vi "TCPClient.vi"() -> ()   [LabVIEW 2014]
uses:
  Global/ClientGlobalCY.vi
  CYY/cyy.lvlib
  LeakageFenxi/LeakageFenXi.lvlib
panel:
  in  "quit":bool
  in  "获取区域信息":bool
  in  "获取采样数据信息":bool
  in  "选项卡控件":enum32{"数据监测界面", "选项卡 2"}(tab)
  in  "数据监测界面":i32(listbox)
  out "区域信息":string[][](array[string])
  out "采样数据":string[][](array[string])
  out "error out":errorcluster caption="错误输出"
  in  "error in (no error)":errorcluster caption="错误输入（无错误）"
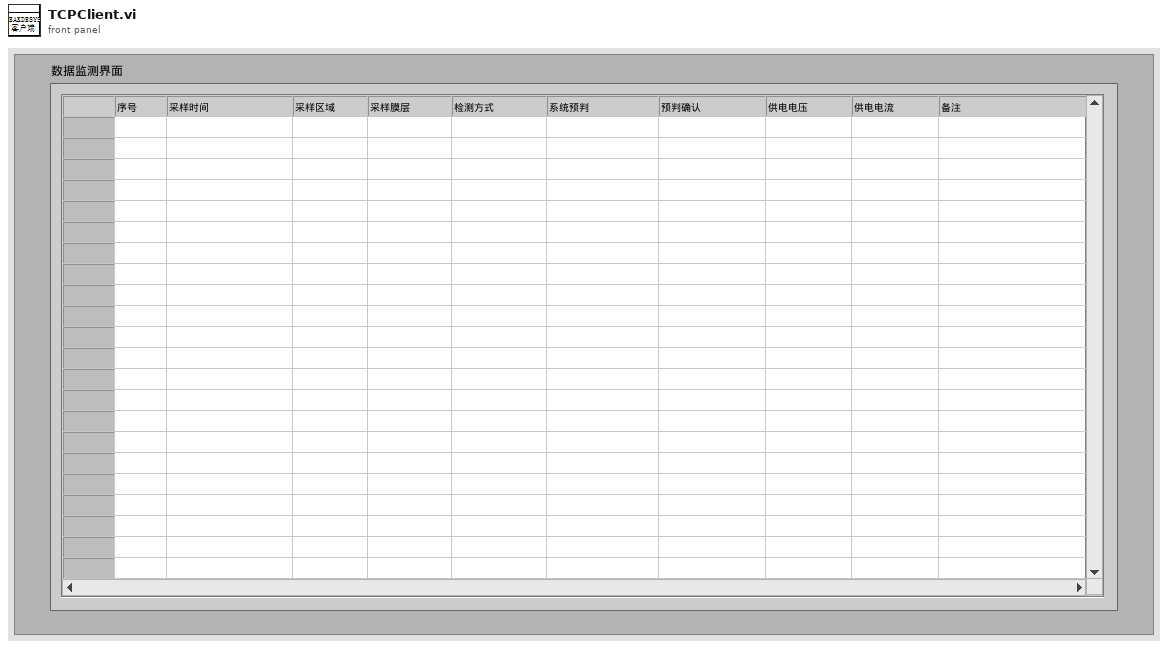
[diagram p1: front panel]
types:
  T1 = enum32{"invalid app kind", "Development System", "Run Time System", "Student Edition", "Embedded LabVIEW", "Evaluation", "Custom"}
  T2 = enum32{"Invalid", "Standard", "Closed", "Hidden", "Minimized", "Maximized"}
  T3 = cluster{"Core":cluster{"Current VI Reference":refnum<vi>, "Close Panel on Exit?":bool}, "Your Boolean data":bool, "Your string data":string, "connectionID":refnum<k5>, "Row":i32, "SampleInfoTime":string, "AreaName":string, "采样数据":string[][], "是否存在记录？":bool}
  T4 = typedef "LVPoint32TypeDef.ctl" = cluster{"Horizontal":i32, "Vertical":i32}
  T5 = typedef "LVRowAndColumnTypeDef.ctl" = cluster{"Row":i32, "Column":i32}
  T6 = typedef "LVRectTypeDef.ctl" = cluster{"Left":i16, "Top":i16, "Right":i16, "Bottom":i16}
  T7 = cluster{"Current VI Reference":refnum<vi>, "Close Panel on Exit?":bool}
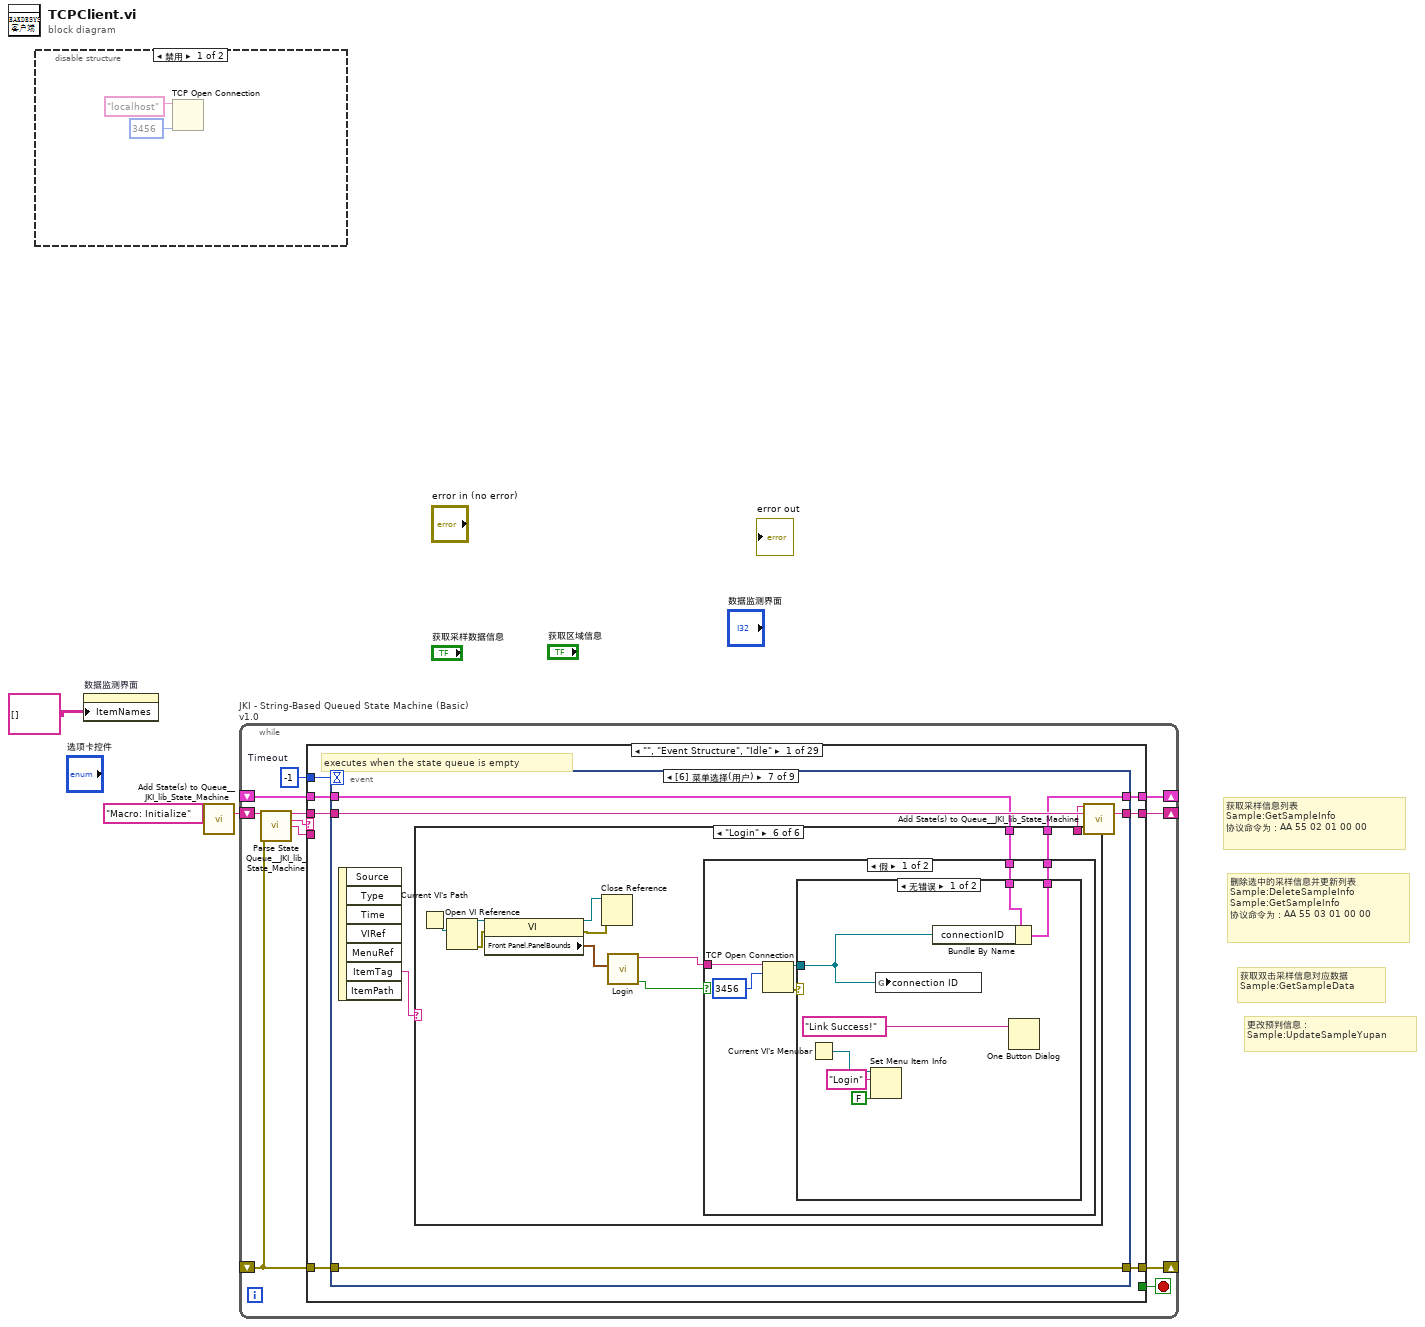
[diagram p0: block diagram]
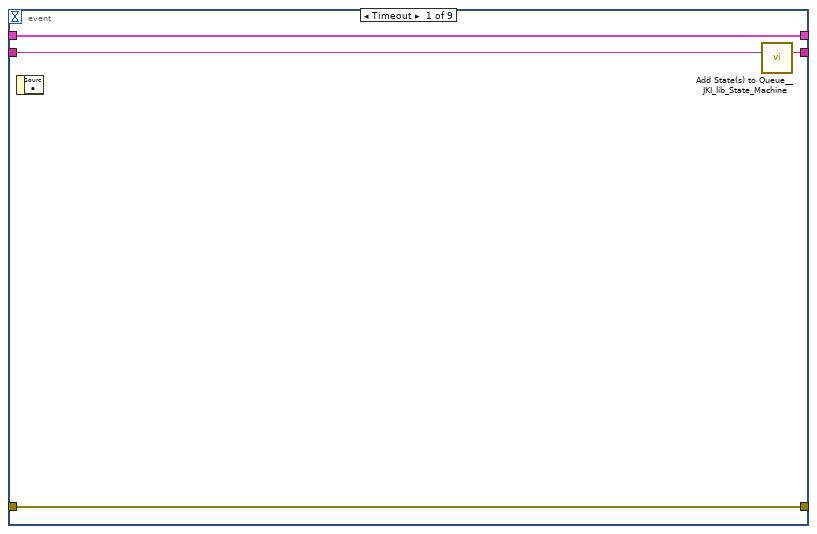
[diagram p3: hidden frame]
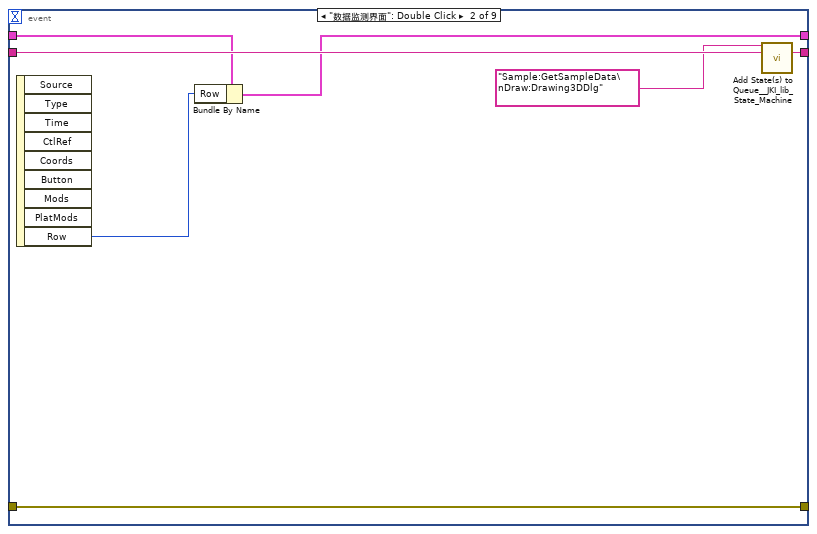
[diagram p4: hidden frame]
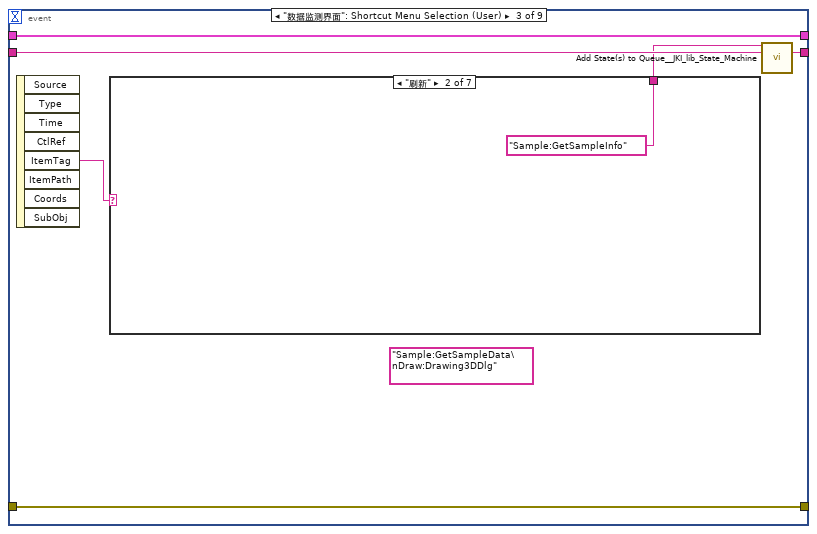
[diagram p5: hidden frame]
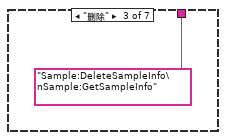
[diagram p7: hidden frame]
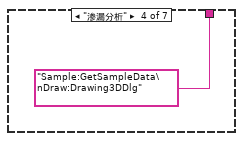
[diagram p8: hidden frame]
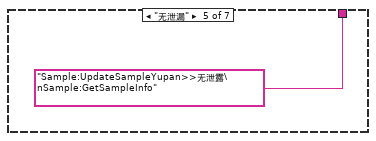
[diagram p9: hidden frame]
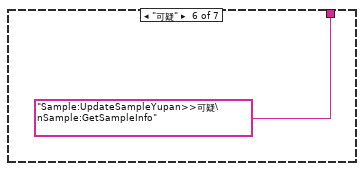
[diagram p10: hidden frame]
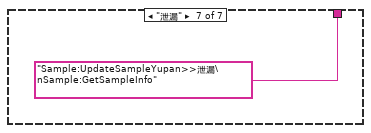
[diagram p11: hidden frame]
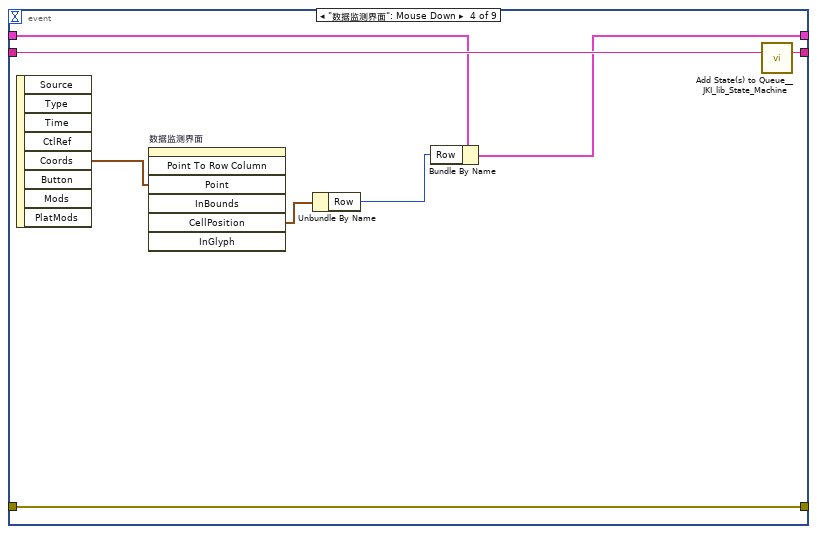
[diagram p12: hidden frame]
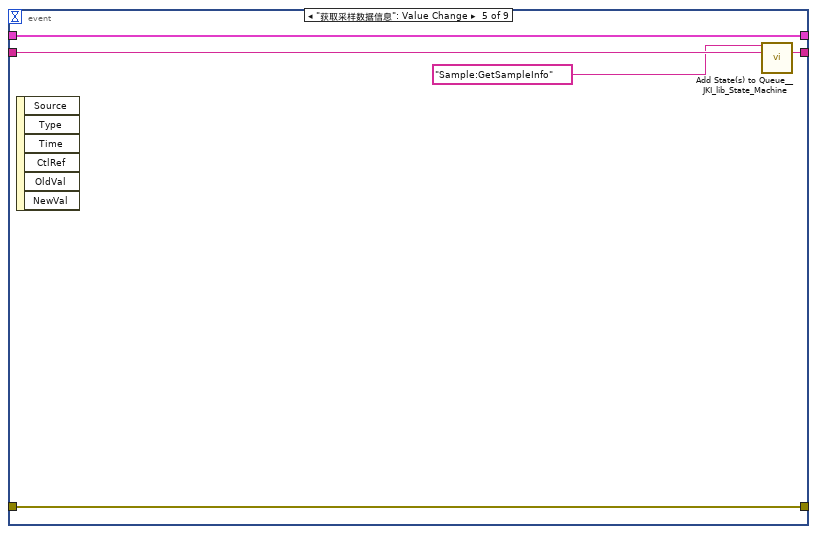
[diagram p13: hidden frame]
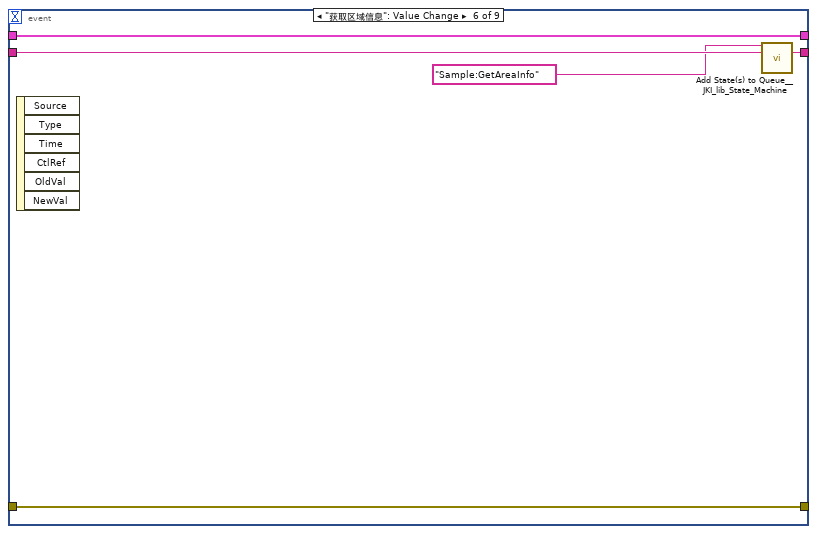
[diagram p14: hidden frame]
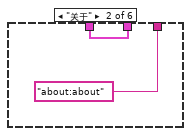
[diagram p16: hidden frame]
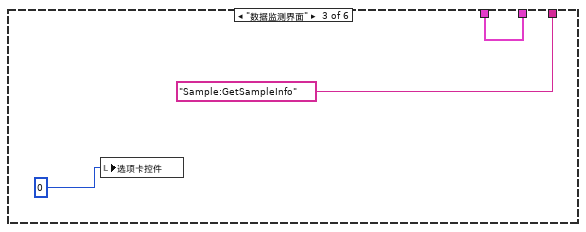
[diagram p17: hidden frame]
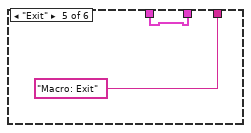
[diagram p19: hidden frame]
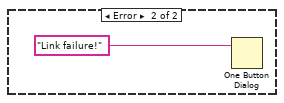
[diagram p20: hidden frame]
diagram:
  # "更改预判信息：\nSample:UpdateSampleYupan"
  # "获取双击采样信息对应数据\nSample:GetSampleData"
  # "删除选中的采样信息并更新列表\nSample:DeleteSampleInfo\nSample:GetSampleInfo\n协议命令为：AA 55 03 01 00 00"
  # "获取采样信息列表\nSample:GetSampleInfo\n协议命令为：AA 55 02 01 00 00"
  n1 = disable-structure shown="禁用" {
    frame Disabled {
      n2 = TCP Open Connection(address="localhost" ("地址"), remote port or service name=u16 3456 ("远程端口或服务名称")) -> ()  [unwired: 3 in, 2 out]
    }
    frame Enabled {
    }
  }
  n3 = property on="数据监测界面" class="MCListbox (严格)"("ItemNames"=string[][] []) -> ()  [unwired: 2 in, 2 out]
  n4 = call <vilib>:"Add State(s) to Queue__JKI_lib_State_Machine.vi"("State(s) in (\"\")"="Macro: Initialize") -> ("States Out"=w3:string)  [unwired: 14 in]
  n5 = while "JKI - String-Based Queued State Machine (Basic) v1.0" {
    shift-right: [w9] -> _
    shift-left: _ -> [w8]
    shift-right: [w12] -> _
    shift-left: _ -> [w6]
    shift-right: [w11] -> _
    shift-left: w3 -> [w13]
    stop <- w10 stop-if-true
    w7 = -1  # Timeout
    n6 = call <vilib>:"Parse State Queue__JKI_lib_State_Machine.vi"("State Queue"=w13, "Error In (no error)"=w6) -> ("Remaining States"=w15:string, "Current State"=w16:string, "Arguments"=w14:string)  [unwired: 11 in]
    n7 = case shown="\"\", \"Event Structure\", \"Idle\"" w16 {
      selector: w16 -> [_ _ w118 _ _ _ _ _ _ _ _ _ _ _ _ _ _ _ _ _ _ _ _ _ _ _ _ _ _]
      tunnel: w15 -> [w23 w117 w122 w140 w146 w151 w155 w168 w174 w178 w182 w188 w199 w225 w230 w240 w244 w248 w252 w256 w260 w264 w272 w276 w291 w308 w320 w327 w334]
      tunnel: w14 -> [_ _ _ _ _ _ _ _ _ _ _ w183 w193 _ _ _ _ _ _ _ _ _ _ _ w280 _ _ _ _]
      tunnel: w8 -> [w21 w114 w120 w131 w143 w149 w152 _ w169 w175 w180 w186 w195 w222 w227 w237 w241 w245 w249 w253 w257 w261 w269 w273 w288 w298 w317 w325 w330]
      tunnel: [w20 w115 w124 w137 errorcluster {"status"=FALSE, "code"=0, "source"=""} ("error out") w148 w153 w165 w170 w176 w179 w184 w196 w223 w228 w238 w242 w246 w250 w254 w258 w262 w270 w274 w289 w306 w318 w322 w331] -> w12
      tunnel: w6 -> [w19 w115 w123 w137 w142 w148 w153 w165 w171 w176 w179 w185 w197 w223 w228 w238 w242 w246 w250 w254 w258 w262 w270 w274 w289 w306 w318 w323 w332]
      tunnel: [w22 w116 w121 w139 w145 w150 w154 w167 w173 w177 w181 w187 w198 w224 w229 w239 w243 w247 w251 w255 w259 w263 w271 w275 w290 w307 w319 w326 w333] -> w11
      tunnel: [_ _ _ _ _ TRUE _ _ _ _ _ _ _ _ _ _ _ _ _ _ _ _ _ _ _ _ _ _ _] -> w10
      tunnel: [w18 w114 w120 w138 w143 w149 w152 w166 w169 w175 w180 w186 w195 w222 w227 w237 w241 w245 w249 w253 w257 w261 w269 w273 w288 w297 w317 w325 w330] -> w9
      tunnel: w7 -> [w17 _ _ _ _ _ _ _ _ _ _ _ _ _ _ _ _ _ _ _ _ _ _ _ _ _ _ _ _]
      frame "", "Event Structure", "Idle" {
        # "executes when the state queue is empty"
        n8 = event shown="[6] 菜单选择(用户)" {
          selector: _ -> [_ _ _ _ _ _ _ _ _]
          dyn-events: _ -> [_ _ _ _ _ _ _ _ _]
          timeout: w17 -> [_ _ _ _ _ _ _ _ _]
          tunnel: w23 -> [w27 w34 w40 w54 w59 w64 w71 w107 w113]
          tunnel: [w26 w33 w39 w53 w58 w63 w70 w106 w112] -> w22
          tunnel: w21 -> [w24 w31 w37 w48 w56 w61 w67 w104 w110]
          tunnel: [w25 w32 w38 w52 w57 w62 w69 w105 w111] -> w20
          tunnel: w19 -> [w25 w32 w38 w52 w57 w62 w69 w105 w111]
          tunnel: [w24 w28 w37 w47 w56 w61 w66 w104 w110] -> w18
          event Timeout {
            n9 = event-data() -> ()  [unwired: 1 in, 1 out]
            n10 = call <vilib>:"Add State(s) to Queue__JKI_lib_State_Machine.vi"("State(s) in (\"\")"=w27) -> ("States Out"=w26:string)  [unwired: 14 in]
          }
          event "数据监测界面": Double Click {
            n11 = event-data() -> ("Row"=w30:i32)  [unwired: 1 in, 8 out]
            n12 = Bundle By Name(cluster=w31, "Row"=w30) -> (w28:T3)
            n13 = call <vilib>:"Add State(s) to Queue__JKI_lib_State_Machine.vi"("State(s) in Front (\"\")"="Sample:GetSampleData\nDraw:Drawing3DDlg", "State(s) in (\"\")"=w34) -> ("States Out"=w33:string)  [unwired: 13 in]
          }
          event "数据监测界面": Shortcut Menu Selection (User) {
            (unwired) "Sample:GetSampleData\nDraw:Drawing3DDlg"
            n14 = event-data() -> ("ItemTag"=w36:string)  [unwired: 1 in, 7 out]
            n15 = case shown="\"刷新\"" w36 {
              tunnel: [_ "Sample:GetSampleInfo" "Sample:DeleteSampleInfo\nSample:GetSampleInfo" "Sample:GetSampleData\nDraw:Drawing3DDlg" "Sample:UpdateSampleYupan>>无泄露\nSample:GetSampleInfo" "Sample:UpdateSampleYupan>>可疑\nSample:GetSampleInfo" "Sample:UpdateSampleYupan>>泄漏\nSample:GetSampleInfo"] -> w35
              frame "假", Default {
              }
              frame "刷新" {
              }
              frame "删除" {
              }
              frame "渗漏分析" {
              }
              frame "无泄漏" {
              }
              frame "可疑" {
              }
              frame "泄漏" {
              }
            }
            n16 = call <vilib>:"Add State(s) to Queue__JKI_lib_State_Machine.vi"("State(s) in Front (\"\")"=w35, "State(s) in (\"\")"=w40) -> ("States Out"=w39:string)  [unwired: 13 in]
          }
          event "数据监测界面": Mouse Down {
            n17 = event-data() -> ("Coords"=w51:T4)  [unwired: 1 in, 7 out]
            n18 = invoke on="数据监测界面" class="MCListbox (严格)" method="Point To Row Column"("Point"=w51) -> ("CellPosition"=w50:T5)  [unwired: 6 in, 6 out]
            n19 = Unbundle By Name(w50) -> ("Row"=w49:i32)
            n20 = Bundle By Name(cluster=w48, "Row"=w49) -> (w47:T3)
            n21 = call <vilib>:"Add State(s) to Queue__JKI_lib_State_Machine.vi"("State(s) in (\"\")"=w54) -> ("States Out"=w53:string)  [unwired: 14 in]
          }
          event "获取采样数据信息": Value Change {
            n22 = event-data() -> ()  [unwired: 1 in, 6 out]
            n23 = call <vilib>:"Add State(s) to Queue__JKI_lib_State_Machine.vi"("State(s) in Front (\"\")"="Sample:GetSampleInfo", "State(s) in (\"\")"=w59) -> ("States Out"=w58:string)  [unwired: 13 in]
          }
          event "获取区域信息": Value Change {
            n24 = event-data() -> ()  [unwired: 1 in, 6 out]
            n25 = call <vilib>:"Add State(s) to Queue__JKI_lib_State_Machine.vi"("State(s) in Front (\"\")"="Sample:GetAreaInfo", "State(s) in (\"\")"=w64) -> ("States Out"=w63:string)  [unwired: 13 in]
          }
          event Menu Selection (User) {
            n26 = event-data() -> ("ItemTag"=w68:string)  [unwired: 1 in, 6 out]
            n27 = case shown="\"Login\"" w68 {
              tunnel: w67 -> [_ w73 w75 _ w78 w80]
              tunnel: [_ w73 w75 _ w78 w79] -> w66
              tunnel: [_ "about:about" "Sample:GetSampleInfo" _ "Macro: Exit" _] -> w65
              frame "假", Default {
              }
              frame "关于" {
              }
              frame "数据监测界面" {
                n28 = local write "选项卡控件"(0) -> ()
              }
              frame "Logout" {
              }
              frame "Exit" {
              }
              frame "Login" {
                n29 = Current VI's Path() -> (path=w88:path)
                n30 = Open VI Reference(vi path=w88) -> (vi reference=w87:refnum<vi>, error out=w86:errorcluster)  [unwired: 5 in]
                n31 = property class="VI"(reference=w87, error in=w86) -> (reference out=w84:refnum<vi>, error out=w85:errorcluster, "Front Panel.PanelBounds"=w83:T6)
                n32 = Close Reference(reference=w84, error in (no error)=w85) -> ()  [unwired: 1 out]
                n33 = call "Login.vi"("窗口边界"=w83) -> ("drop?"=w82:bool, "User IP"=w81:string)  [unwired: 8 in, 1 out]
                n34 = case shown="假" w82 {
                  tunnel: w81 -> [w94 _]
                  tunnel: w80 -> [w90 _]
                  tunnel: [w89 _] -> w79
                  frame False {
                    n35 = TCP Open Connection(address=w94, remote port or service name=u16 3456 ("远程端口或服务名称")) -> (connection ID=w91:refnum<k5>, error out=w92:errorcluster)  [unwired: 3 in]
                    n36 = case shown="无错误" w92 {
                      tunnel: w91 -> [w95 _]
                      tunnel: w90 -> [w97 _]
                      tunnel: [w96 _] -> w89
                      frame No Error {
                        n37 = Current VI's Menubar() -> (w101:refnum<k9>)
                        n38 = Set Menu Item Info(7:"Login" ("项名称"), 9:FALSE ("已启用"), 11:w101) -> ()  [unwired: 4 in, 2 out]
                        n39 = global write "ClientGlobalCY.vi" "connection ID"(w95) -> ()
                        n40 = Bundle By Name(cluster=w97, "connectionID"=w95) -> (w96:T3)
                        n41 = One Button Dialog(message="Link Success!" ("消息")) -> ()  [unwired: 1 in, 1 out]
                      }
                      frame Error {
                        n42 = One Button Dialog(message="Link failure!" ("消息")) -> ()  [unwired: 1 in, 1 out]
                      }
                    }
                  }
                  frame True {
                  }
                }
              }
            }
            n43 = call <vilib>:"Add State(s) to Queue__JKI_lib_State_Machine.vi"("State(s) in Front (\"\")"=w65, "State(s) in (\"\")"=w71) -> ("States Out"=w70:string)  [unwired: 13 in]
          }
          event "quit": Value Change {
            n44 = event-data() -> ()  [unwired: 1 in, 1 out]
            n45 = call <vilib>:"Add State(s) to Queue__JKI_lib_State_Machine.vi"("State(s) in Front (\"\")"="Macro: Exit", "State(s) in (\"\")"=w107) -> ("States Out"=w106:string)  [unwired: 13 in]
          }
          event Panel Close? {
            # "Discard the event because we'll close the front panel ourselves in Macro: Exit"
            # "Close Panel button (pressed) Event\n(this executes Macro: Exit to terminate the VI)"
            n46 = event-data() -> ()  [unwired: 1 in, 1 out]
            n47 = event-data("Discard?"=TRUE) -> ()  [unwired: 1 in, 1 out]
            n48 = call <vilib>:"Add State(s) to Queue__JKI_lib_State_Machine.vi"("State(s) in Front (\"\")"="Macro: Exit", "State(s) in (\"\")"=w113) -> ("States Out"=w112:string)  [unwired: 13 in]
          }
        }
      }
      frame "---------- Core ----------" {
        # "Do not put any code in this frame.\n(it is a separator no-op)"
        n49 = call <vilib>:"Add State(s) to Queue__JKI_lib_State_Machine.vi"("State(s) in (\"\")"=w117) -> ("States Out"=w116:string)  [unwired: 14 in]
      }
      frame Default {
        w127 = 42 items=["No error", "Argument error", "Memory is full", "Out of zone", "End of file", "File already open", "Generic file I/O error", "File not found", "File permission error", "Disk is full", "Duplicate path", "Too many files open", "System feature not enabled", "Resource file not found", "Cannot add resource", "Resource not found", "Image not found", "Image memory error", "Pen does not exist", "Config type invalid", "Config token not found", "Config parse error", "Config memory error", "Bad external code format", "Bad external code offset", "External code not present", "Null window", "Destroy window error", "Null menu", "Print aborted", "Bad print record", "Print driver error", "Windows error during printing", "Memory error during printing", "Print dialog error", "Generic print error", "Invalid device refnum", "Device not found", "Device parameter error", "Device unit error", "Cannot open device", "Device call aborted", "Generic error", "Cancelled by user", "Object ID too low", "Object ID too high", "Object not in heap", "Unknown heap", "Unknown object (invalid DefProc)", "Unknown object (DefProc not in table)", "Message out of range", "Invalid (null) method", "Unknown message", "Manager call not supported", "Bad address", "Network operation in progress", "Network operation timed out", "Connection is busy", "Network attribute not supported", "Network error", "Address in use", "System out of memory", "Connection aborted", "Connection refused", "Not connected", "Already connected", "Connection closed", "Initialization error (interapplication manager)", "Bad occurrence", "Wait on unbound occurrence handler", "Occurrence queue overflow", "Datalog type conflict", "Unused", "Unrecognized type (interapplication manager)", "Memory corrupt", "Failed to make temporary DLL", "Old CIN version", "Drag socket not found", "Failed to load drop-object", "Failed to register OLE object", "Failed to release OLE object", "Format specifier type mismatch", "Unknown format specifier", "Too few format specifiers", "Too many format specifiers", "Scan failed", "Newer CIN version", "Error converting to variant", "Runtime menu error", "Password tampered", "Variant attribute not found", "Incompatible variant data type", "Event data is not available", "Event Store is not present", "Occurrence is not found", "Event Queue is not created", "Event info is not available", "Refnum passed is NULL", "Error retrieving Class GUID", "Error retrieving CoClass GUID", "Error retrieving TypeLib GUID.", "Bad built application magic bytes.", "Specific driver is different from the specific driver associated with the Logical Name.", "There is no session opened to the class driver.", "Max Error", "MAX - Error with config objects", "MAX - Error loading configuration", "MAX - Group not supported"]
        # "Current State"
        # "Do not delete, rename, or modify this frame.\n(this is used to capture unhandled states and typos)"
        # "Handle mistyped state name (developer tool)"
        n50 = Format Into String(format string="Software Exception: Unhandled State \"%s\"." ("message"), error in=w123, w118) -> (resulting string=w126:string, error out=w125:errorcluster)  [unwired: 1 in]
        n51 = call <vilib>:"Error Cluster From Error Code.vi"("show call chain? (False)"=TRUE, "error in (no error)"=w125, "error message (\"\")"=w126, "error code (0)"=w127) -> ("error out"=w124:errorcluster)  [unwired: 5 in]
        n52 = call <vilib>:"Add State(s) to Queue__JKI_lib_State_Machine.vi"("State(s) in (\"\")"=w122) -> ("States Out"=w121:string)  [unwired: 14 in]
      }
      frame "Initialize Core Data" {
        # "Do not delete, rename, or modify this frame.\n(this is used to determine panel behavior on exit)"
        # "originally closed?"
        # "exe?"
        # "If panel starts closed or is an EXE, then close it when we exit"
        n53 = property class="VI"() -> ("Front Panel.Open"=w136:bool)  [unwired: 2 in, 2 out]
        n54 = property class="App"() -> ("App.Kind"=w135:T1)  [unwired: 2 in, 2 out]
        n55 = control-ref of="Current VI Reference"() -> (w129:refnum<vi>)
        n56 = Not(x=w136) -> (.not. x?=w133:bool)
        n57 = Equal?(x=w135, y=T1."Run Time System" ("Application:Kind")) -> (x = y?=w132:bool)
        n58 = Or(x=w133, y=w132) -> (x .or. y?=w130:bool)
        n59 = Bundle By Name(cluster=w131, "Core.Current VI Reference"=w129, "Core.Close Panel on Exit?"=w130) -> (w138:T3)
        n60 = call <vilib>:"Add State(s) to Queue__JKI_lib_State_Machine.vi"("State(s) in (\"\")"=w140) -> ("States Out"=w139:string)  [unwired: 14 in]
      }
      frame "Error Handler" {
        # "Unhandled Error -- Display it"
        # "Handle any errors here.\nYou can also output any states to clean-up after errors occur"
        # "Clear error"
        n61 = call <vilib>:"General Error Handler.vi"("error in (no error)"=w142) -> ()  [unwired: 10 in, 5 out]
        n62 = call <vilib>:"Add State(s) to Queue__JKI_lib_State_Machine.vi"("State(s) in Front (\"\")"="/* Post Error States", "State(s) in (\"\")"=w146) -> ("States Out"=w145:string)  [unwired: 13 in]
      }
      frame "Exit" {
        # "Do not put any code in this frame.\n(No errors that occur here will be handled.)"
        n63 = call <vilib>:"Add State(s) to Queue__JKI_lib_State_Machine.vi"("State(s) in (\"\")"=w151) -> ("States Out"=w150:string)  [unwired: 14 in]
      }
      frame "---------- Data ----------" {
        # "Do not put any code in this frame.\n(It is a separator no-op. You can make a copy of this frame to create a new Data frame)"
        n64 = call <vilib>:"Add State(s) to Queue__JKI_lib_State_Machine.vi"("State(s) in (\"\")"=w155) -> ("States Out"=w154:string)  [unwired: 14 in]
      }
      frame "Data: Initialize" {
        w156 = TRUE  # 是否存在记录？
        w158 = ""  # AreaName
        w159 = ""  # SampleInfoTime
        w160 = 0  # Row
        w161 = refnum<k5> refnum  # connectionID
        w162 = T7 {"Current VI Reference"=refnum, "Close Panel on Exit?"=FALSE}  # Core
        w164 = TRUE  # Your Boolean data
        w163 = ""  # Your string data
        # "do not delete - used by framework"
        # "Data names and types of shift register data are defined by this bundle."
        # "Initialize the shift-register data, here.\n(data names are defined by what you wire into the bundle function)"
        n65 = Bundle("Core"=w162, "Your Boolean data"=w164, "Your string data"=w163, "connectionID"=w161, "Row"=w160, "SampleInfoTime"=w159, "AreaName"=w158, "采样数据"=string[][] [["101", "39", "0", "9.701"], ["102", "37", "0", "9.699"], ["103", "40", "2", "9.699"], ["104", "38", "2", "9.696"], ["105", "36", "2", "9.698"], ["106", "41", "4", "9.708"], ["107", "39", "4", "9.699"], ["108", "37", "4", "9.702"], ["109", "35", "4", "9.703"], ["110", "40", "6", "9.698"], ["111", "36", "6", "9.690"], ["112", "41", "8", "9.707"], ["113", "39", "8", "9.705"], ["114", "37", "8", "9.694"], ["115", "35", "8", "9.698"], ["116", "40", "10", "9.702"], ["117", "38", "10", "9.703"], ["118", "36", "10", "9.699"], ["119", "34", "10", "9.700"], ["120", "39", "12", "9.704"], ["121", "37", "12", "9.699"], ["122", "40", "14", "9.700"], ["123", "38", "14", "9.699"], ["124", "36", "14", "9.699"], ["125", "41", "16", "9.699"], ["126", "39", "16", "9.698"], ["127", "37", "16", "9.701"], ["128", "35", "16", "9.696"], ["129", "40", "18", "9.697"], ["130", "36", "17.75", "9.698"], ["131", "70", "0", "9.701"], ["132", "60", "0", "9.700"], ["133", "50", "0", "9.701"], ["134", "40", "8", "9.699"], ["135", "32", "8", "9.699"], ["136", "40", "0", "9.696"], ["137", "32", "0", "9.698"], ["138", "40", "8", "9.708"], ["139", "32", "8", "9.699"], ["140", "40", "0", "9.702"], ["141", "70", "0", "9.703"], ["142", "60", "0", "9.698"], ["201", "33", "0", "9.690"], ["202", "31", "0", "9.707"], ["203", "34", "2", "9.705"], ["204", "32", "2", "9.694"], ["205", "30", "2", "9.698"], ["206", "28", "2", "9.702"], ["207", "33", "4", "9.703"], ["208", "31", "4", "9.699"], ["209", "29", "4", "9.700"], ["210", "27", "4", "9.704"], ["211", "34", "6", "9.699"], ["212", "30", "6", "9.700"], ["213", "28", "6", "9.699"], ["214", "33", "8", "9.699"], ["215", "31", "8", "9.699"], ["216", "29", "8", "9.698"], ["217", "27", "8", "9.701"], ["218", "32", "10", "9.696"], ["219", "30", "10", "9.697"], ["220", "28", "10", "9.698"], ["221", "33", "12", "9.701"], ["222", "31", "12", "9.700"], ["223", "34", "14", "9.701"], ["224", "32", "14", "9.699"], ["225", "30", "14", "9.699"], ["226", "28", "14", "9.696"], ["227", "33", "16", "9.698"], ["228", "31", "16", "9.708"], ["229", "29", "16", "9.699"], ["230", "34", "17.5", "9.702"], ["231", "30", "17", "9.703"], ["232", "28", "17", "9.698"], ["233", "40", "0", "9.690"], ["234", "30", "0", "9.707"], ["235", "24", "8", "9.705"], ["236", "16", "8", "9.694"], ["237", "24", "0", "9.698"], ["238", "16", "0", "9.702"], ["239", "24", "8", "9.703"], ["240", "32", "0", "9.699"], ["241", "24", "0", "9.700"], ["242", "16", "0", "9.704"], ["243", "50", "0", "9.699"], ["244", "40", "0", "9.700"], ["245", "30", "0", "9.699"], ["301", "27", "0", "9.699"], ["302", "25", "0", "9.699"], ["303", "21", "0", "9.698"], ["304", "19", "0", "9.701"], ["305", "26", "2", "9.696"], ["306", "24", "2", "9.697"], ["307", "22", "2", "9.698"], ["308", "20", "2", "9.701"], ["309", "18", "2", "9.700"], ["310", "25", "4", "9.701"], ["311", "23", "4", "9.699"], ["312", "21", "4", "9.699"], ["313", "19", "4", "9.696"], ["314", "17", "4", "9.698"], ["315", "24", "6", "9.708"], ["316", "22", "6", "9.699"], ["317", "18", "6", "9.702"], ["318", "25", "8", "9.703"], ["319", "23", "8", "9.698"], ["320", "21", "8", "9.690"], ["321", "19", "8", "9.707"], ["322", "26", "10", "9.705"], ["323", "24", "10", "9.694"], ["324", "22", "10", "9.698"], ["325", "20", "10", "9.702"], ["326", "18", "10", "9.703"], ["327", "27", "12", "9.699"], ["328", "25", "12", "9.700"], ["329", "21", "12", "9.704"], ["330", "19", "12", "9.699"], ["331", "26", "14", "9.700"], ["332", "24", "14", "9.699"], ["333", "22", "14", "9.699"], ["334", "20", "14", "9.699"], ["335", "27", "16", "9.698"], ["336", "25", "16", "9.701"], ["337", "23", "16", "9.696"], ["338", "21", "16", "9.697"], ["339", "19", "16", "9.698"], ["340", "24", "17", "9.701"], ["341", "22", "17", "9.700"], ["342", "18", "17.5", "9.701"], ["401", "15", "0", "9.699"], ["402", "13", "0", "9.699"], ["403", "16", "2", "9.696"], ["404", "14", "2", "9.698"], ["405", "12", "2", "9.708"], ["406", "15", "4", "9.699"], ["407", "13", "4", "9.702"], ["408", "11", "4", "9.703"], ["409", "16", "6", "9.698"], ["410", "12", "6", "9.690"], ["411", "47", "8", "9.707"], ["412", "15", "8", "9.705"], ["413", "13", "8", "9.694"], ["414", "11", "8", "9.698"], ["415", "16", "10", "9.702"], ["416", "14", "10", "9.703"], ["417", "12", "10", "9.699"], ["418", "10", "10", "9.700"], ["419", "15", "12", "9.704"], ["420", "13", "12", "9.699"], ["421", "18", "14", "9.700"], ["422", "16", "14", "9.699"], ["423", "14", "14", "9.699"], ["424", "12", "14", "9.699"], ["425", "17", "16", "9.698"], ["426", "15", "16", "9.701"], ["427", "13", "16", "9.696"], ["428", "16", "17.5", "9.697"], ["429", "12", "18", "9.698"], ["430", "10", "18", "9.701"], ["431", "30", "0", "9.700"], ["432", "20", "0", "9.701"], ["433", "0", "0", "9.699"], ["434", "8", "0", "9.699"], ["435", "0", "0", "9.696"], ["436", "16", "8", "9.698"], ["437", "8", "8", "9.708"], ["438", "0", "8", "9.699"], ["439", "20", "0", "9.702"], ["440", "10", "0", "9.703"], ["441", "0", "0", "9.698"], ["501", "10", "2", "9.690"], ["502", "8", "2", "9.707"], ["503", "6", "2", "9.705"], ["504", "4", "2", "9.694"], ["505", "2", "2", "9.698"], ["506", "0", "2", "9.702"], ["507", "9", "4", "9.703"], ["508", "7", "4", "9.699"], ["509", "5", "4", "9.700"], ["510", "3", "4", "9.704"], ["511", "1", "4", "9.699"], ["512", "10", "6", "9.700"], ["513", "6", "6", "9.699"], ["514", "4", "6", "9.699"], ["515", "2", "6", "9.699"], ["516", "0", "6", "9.698"], ["517", "9", "8", "9.701"], ["518", "7", "8", "9.696"], ["519", "5", "8", "9.697"], ["520", "3", "8", "9.698"], ["521", "1", "8", "9.701"], ["522", "8", "10", "9.700"], ["523", "6", "10", "9.701"], ["524", "4", "10", "9.699"], ["525", "2", "10", "9.699"], ["526", "0", "10", "9.696"], ["527", "9", "12", "9.698"], ["528", "7", "12", "9.708"], ["529", "3", "12", "9.699"], ["530", "1", "12", "9.702"], ["531", "0", "18", "9.703"], ["532", "10", "14", "9.698"], ["533", "8", "14", "9.690"], ["534", "6", "14", "9.707"], ["535", "4", "14", "9.705"], ["536", "2", "14", "9.694"], ["537", "0", "14", "9.698"], ["538", "11", "16", "9.702"], ["539", "9", "16", "9.703"], ["540", "7", "16", "9.699"], ["541", "5", "16", "9.700"], ["542", "3", "16", "9.704"], ["543", "1", "16", "9.699"], ["544", "6", "18", "9.700"], ["545", "4", "18", "9.699"]], "是否存在记录？"=w156) -> (w166:T3)  [unwired: 1 in]
        n66 = call <vilib>:"Add State(s) to Queue__JKI_lib_State_Machine.vi"("State(s) in (\"\")"=w168) -> ("States Out"=w167:string)  [unwired: 14 in]
      }
      frame "Data: Cleanup" {
        # "Cleanup any data and references, here.\n(this is called automatically, by the Macro: Exit)"
        n67 = Unbundle By Name(w169) -> ("Core.Current VI Reference"=w172:refnum<vi>)
        n68 = Close Reference(reference=w172, error in (no error)=w171) -> (error out=w170:errorcluster)
        n69 = call <vilib>:"Add State(s) to Queue__JKI_lib_State_Machine.vi"("State(s) in (\"\")"=w174) -> ("States Out"=w173:string)  [unwired: 14 in]
      }
      frame "---------- UI ----------" {
        # "Do not put any code in this frame.\n(It is a separator no-op. You can make a copy of this frame to create a new UI frame)"
        n70 = call <vilib>:"Add State(s) to Queue__JKI_lib_State_Machine.vi"("State(s) in (\"\")"=w178) -> ("States Out"=w177:string)  [unwired: 14 in]
      }
      frame "UI: Initialize" {
        # "Initialize the User Interface, here.\n(this is called automatically, by the Macro: Init)"
        n71 = call <vilib>:"Add State(s) to Queue__JKI_lib_State_Machine.vi"("State(s) in (\"\")"=w182) -> ("States Out"=w181:string)  [unwired: 14 in]
      }
      frame "UI: Cursor Set" {
        # "Argument"
        # "Set and Unset Cursor Busy.\n(Usage: \"UI: Cursor Set >> Busy|Idle\")"
        n72 = case shown="\"Idle\", 默认" w183 {
          tunnel: w185 -> [w190 w192]
          tunnel: [w189 w191] -> w184
          frame "Idle", Default {
            n73 = call <vilib>:"Unset Busy.vi"("error in (no error)"=w190) -> ("error out"=w189:errorcluster)  [unwired: 10 in]
          }
          frame "Busy" {
            n74 = call <vilib>:"Set Busy.vi"("error in (no error)"=w192) -> ("error out"=w191:errorcluster)  [unwired: 9 in, 1 out]
          }
        }
        n75 = call <vilib>:"Add State(s) to Queue__JKI_lib_State_Machine.vi"("State(s) in (\"\")"=w188) -> ("States Out"=w187:string)  [unwired: 14 in]
      }
      frame "UI: Front Panel State" {
        # "Argument"
        # "Set Front Panel Open or Closed\n(Usage: \"UI: Front Panel State >> Open|Close\")"
        n76 = Unbundle By Name(w195) -> ("Core.Current VI Reference"=w194:refnum<vi>)
        n77 = case shown="\"Open\", 默认" w193 {
          tunnel: w197 -> [w203 w216]
          tunnel: [w205 w217] -> w196
          tunnel: w194 -> [w204 w214]
          frame "Open", Default {
            n78 = property class="VI"(reference=w204, error in=w203) -> (reference out=w201:refnum<vi>, error out=w202:errorcluster, "Front Panel.Open"=w200:bool)
            n79 = case shown="假" w200 {
              tunnel: [w208 w211] -> w205
              tunnel: w202 -> [w207 w211]
              tunnel: w201 -> [w206 _]
              frame False {
                n80 = invoke class="VI" method="FP.Open"(reference=w206, error in=w207, "Activate"=TRUE, "State"=T2."Standard") -> (error out=w208:errorcluster)  [unwired: 1 in, 4 out]
              }
              frame True {
              }
            }
          }
          frame "Close" {
            n81 = property class="VI"(reference=w214, error in=w216) -> (reference out=w213:refnum<vi>, error out=w215:errorcluster, "Front Panel.Open"=w212:bool)
            n82 = case shown="真" w212 {
              tunnel: [w218 w221] -> w217
              tunnel: w215 -> [w218 w220]
              tunnel: w213 -> [_ w219]
              frame False {
              }
              frame True {
                n83 = invoke class="VI" method="FP.Close"(reference=w219, error in=w220) -> (error out=w221:errorcluster)  [unwired: 1 in, 2 out]
              }
            }
          }
        }
        n84 = call <vilib>:"Add State(s) to Queue__JKI_lib_State_Machine.vi"("State(s) in (\"\")"=w199) -> ("States Out"=w198:string)  [unwired: 14 in]
      }
      frame "---------- Macro ----------" {
        # "Do not put any code in this frame.\n(It is a separator no-op. You can make a copy of this frame to create a new Macro frame)"
        n85 = call <vilib>:"Add State(s) to Queue__JKI_lib_State_Machine.vi"("State(s) in (\"\")"=w225) -> ("States Out"=w224:string)  [unwired: 14 in]
      }
      frame "Macro: Initialize" {
        w226 = "Data: Initialize\nInitialize Core Data\nUI: Initialize\nUI: Front Panel State >> Open"  # Data: Initialize Initialize Core Data UI: Initialize UI: Front Panel State >> Open
        # "Initialization Macro\n(This is called once, when the VI starts)"
        n86 = call <vilib>:"Add State(s) to Queue__JKI_lib_State_Machine.vi"("State(s) in Front (\"\")"=w226, "State(s) in (\"\")"=w230) -> ("States Out"=w229:string)  [unwired: 13 in]
      }
      frame "Macro: Exit" {
        # "Exit Macro\n(This is called once, when the VI exits)"
        n87 = Unbundle By Name(w237) -> ("Core.Close Panel on Exit?"=w236:bool)
        n88 = Select(t="UI: Front Panel State >> Close", s=w236, f="") -> (s? t:f=w233:string)
        n89 = call <vilib>:"Add State(s) to Queue__JKI_lib_State_Machine.vi"("State(s) in (\"\")"=w233, "State(s) at Back (\"\")"="Data: Cleanup\nExit") -> ("States Out"=w231:string)  [unwired: 13 in]
        n90 = call <vilib>:"Add State(s) to Queue__JKI_lib_State_Machine.vi"("State(s) in Front (\"\")"=w231, "State(s) in (\"\")"=w240) -> ("States Out"=w239:string)  [unwired: 13 in]
      }
      frame "---------- New Category ----------" {
        # "Template Separator\n(You can make a copy of, or modify, this frame)"
        n91 = call <vilib>:"Add State(s) to Queue__JKI_lib_State_Machine.vi"("State(s) in (\"\")"=w244) -> ("States Out"=w243:string)  [unwired: 14 in]
      }
      frame "New Category: 1" {
        # "Your code here.\n(You can make a copy of, or modify, this frame)"
        n92 = call <vilib>:"Add State(s) to Queue__JKI_lib_State_Machine.vi"("State(s) in (\"\")"=w248) -> ("States Out"=w247:string)  [unwired: 14 in]
      }
      frame "New Category: 2" {
        # "Your code here.\n(You can make a copy of, or modify, this frame)"
        n93 = call <vilib>:"Add State(s) to Queue__JKI_lib_State_Machine.vi"("State(s) in (\"\")"=w252) -> ("States Out"=w251:string)  [unwired: 14 in]
      }
      frame "---------about--------" {
        # "Your code here.\n(You can make a copy of, or modify, this frame)"
        n94 = call <vilib>:"Add State(s) to Queue__JKI_lib_State_Machine.vi"("State(s) in (\"\")"=w256) -> ("States Out"=w255:string)  [unwired: 14 in]
      }
      frame "about:about" {
        # "Your code here.\n(You can make a copy of, or modify, this frame)"
        n95 = call "HelpDlg.vi"() -> ()  [unwired: 12 in]
        n96 = call <vilib>:"Add State(s) to Queue__JKI_lib_State_Machine.vi"("State(s) in (\"\")"=w260) -> ("States Out"=w259:string)  [unwired: 14 in]
      }
      frame "--------Drawing-------" {
        # "Your code here.\n(You can make a copy of, or modify, this frame)"
        n97 = call <vilib>:"Add State(s) to Queue__JKI_lib_State_Machine.vi"("State(s) in (\"\")"=w264) -> ("States Out"=w263:string)  [unwired: 14 in]
      }
      frame "Draw:Drawing3DDlg" {
        # "Your code here.\n(You can make a copy of, or modify, this frame)"
        n98 = Unbundle By Name(w269) -> ("采样数据"=w266:string[][], "SampleInfoTime"=w265:string, "是否存在记录？"=w267:bool)  [unwired: 1 out]
        n99 = call "IndexSampleData.vi"("SampleData"=w266) -> ("SampleDataXYZ"=w268:cluster{"X":dbl[], "Y":dbl[], "Z":dbl[]})  [unwired: 7 in, 3 out]
        n100 = call "LeakageFenxi.vi"("采样时间"=w265, "Area_name"=w265, "采样数据"=w266, "是否存在记录"=w267, "3DData"=w268) -> ()  [unwired: 7 in]
        n101 = call <vilib>:"Add State(s) to Queue__JKI_lib_State_Machine.vi"("State(s) in (\"\")"=w272) -> ("States Out"=w271:string)  [unwired: 14 in]
      }
      frame "--------Sample---------" {
        # "Your code here.\n(You can make a copy of, or modify, this frame)"
        n102 = call <vilib>:"Add State(s) to Queue__JKI_lib_State_Machine.vi"("State(s) in (\"\")"=w276) -> ("States Out"=w275:string)  [unwired: 14 in]
      }
      frame "Sample:UpdateSampleYupan" {
        # "Your code here.\n(You can make a copy of, or modify, this frame)"
        n103 = property on="数据监测界面" class="MCListbox (严格)"() -> ("ItemNames"=w284:string[][])  [unwired: 2 in, 2 out]
        n104 = Unbundle By Name(w288) -> ("connectionID"=w277:refnum<k5>, "Row"=w283:i32)
        n105 = Index Array(array=w284, index (row)=w283) -> (element=w287:string[])  [unwired: 1 in]
        n106 = Index Array(array=w287, index=1) -> (element=w281:string)
        n107 = Index Array(array=w287, index=0) -> (element=w282:string)
        n108 = call "UpdateSampleYupanInfo.vi"("TCP网络连接输入"=w277, "预判信息"=w280, "Row"=w283, "id"=w282, "SampleTime"=w281) -> ("成功?"=w279:bool)  [unwired: 9 in, 1 out]
        n109 = case shown="真" w279 {
          tunnel: [_ "Sample:GetSampleInfo"] -> w278
          frame False {
          }
          frame True {
          }
        }
        n110 = call <vilib>:"Add State(s) to Queue__JKI_lib_State_Machine.vi"("State(s) in Front (\"\")"=w278, "State(s) in (\"\")"=w291) -> ("States Out"=w290:string)  [unwired: 13 in]
      }
      frame "Sample:GetSampleData" {
        # "Your code here.\n(You can make a copy of, or modify, this frame)"
        n111 = Unbundle By Name(w298) -> ("Row"=w299:i32)  [unwired: 1 out]
        n112 = property on="数据监测界面" class="MCListbox (严格)"() -> ("ItemNames"=w303:string[][])  [unwired: 2 in, 2 out]
        n113 = Index Array(array=w303, index (row)=w299) -> (element=w301:string[])  [unwired: 1 in]
        n114 = Index Array(array=w301, index=0) -> (element=w294:string)
        n115 = Index Array(array=w301, index=1 ("索引")) -> (element=w293:string)
        n116 = Index Array(array=w301, index=2) -> (element=w302:string)
        n117 = call "GetSampleData.vi"("id"=w294, "SampleTime"=w293) -> ("采样数据"=w296:string[][], "存在记录？"=w295:bool)  [unwired: 11 in, 1 out]
        "采样数据" <- w296
        n118 = Bundle By Name(cluster=w298, "SampleInfoTime"=w293, "AreaName"=w302, "采样数据"=w296, "是否存在记录？"=w295) -> (w297:T3)
        n119 = call <vilib>:"Add State(s) to Queue__JKI_lib_State_Machine.vi"("State(s) in (\"\")"=w308) -> ("States Out"=w307:string)  [unwired: 14 in]
      }
      frame "Sample:DeleteSampleInfo" {
        # "Your code here.\n(You can make a copy of, or modify, this frame)"
        n120 = Unbundle By Name(w317) -> ("connectionID"=w309:refnum<k5>, "Row"=w315:i32)
        n121 = property on="数据监测界面" class="MCListbox (严格)"() -> ("ItemNames"=w316:string[][])  [unwired: 2 in, 2 out]
        n122 = Index Array(array=w316, index (row)=w315) -> (element=w314:string[])  [unwired: 1 in]
        n123 = Index Array(array=w314, index=1) -> (element=w310:string)
        n124 = Index Array(array=w314, index=0) -> (element=w311:string)
        n125 = call "DeleteSampleInfo.vi"("TCP网络连接输入"=w309, "Row"=w315, "id"=w311, "SampleTime"=w310) -> ()  [unwired: 10 in, 2 out]
        n126 = call <vilib>:"Add State(s) to Queue__JKI_lib_State_Machine.vi"("State(s) in (\"\")"=w320) -> ("States Out"=w319:string)  [unwired: 14 in]
      }
      frame "Sample:GetSampleInfo" {
        # "Your code here.\n(You can make a copy of, or modify, this frame)"
        n127 = Unbundle By Name(w325) -> ("connectionID"=w324:refnum<k5>)
        n128 = call "GetSampleInfo.vi"("TCP网络连接输入"=w324, "错误输入（无错误）"=w323) -> ("值"=w321:string[][], "错误输出"=w322:errorcluster)  [unwired: 10 in, 2 out]
        n129 = property on="数据监测界面" class="MCListbox (严格)"("ItemNames"=w321) -> ()  [unwired: 2 in, 2 out]
        n130 = call <vilib>:"Add State(s) to Queue__JKI_lib_State_Machine.vi"("State(s) in (\"\")"=w327) -> ("States Out"=w326:string)  [unwired: 14 in]
      }
      frame "Sample:GetAreaInfo" {
        # "Your code here.\n(You can make a copy of, or modify, this frame)"
        n131 = control-ref of="区域信息"() -> (w329:refnum<vi>)
        n132 = call "GetAreaInfo.vi"("reference"=w329, "错误输入（无错误）"=w332) -> ("值"=→"区域信息":string[][], "错误输出"=w331:errorcluster)  [unwired: 12 in]
        n133 = call <vilib>:"Add State(s) to Queue__JKI_lib_State_Machine.vi"("State(s) in (\"\")"=w334) -> ("States Out"=w333:string)  [unwired: 14 in]
      }
    }
  }
